vi "Update time.vi"(8 "error in (no error)":errorcluster, 10 "Time Stamp Control":timestamp, 11 "Common Measurements Interface in":refnum<class "Common Measurements Interface.lvclass">) -> (0 "error out":errorcluster, 3 "Common Measurements Interface out":refnum<class "Common Measurements Interface.lvclass">)   [LabVIEW 2015, in "Common Measurements Interface.lvclass"]
uses:
  Common Measurements Interface.lvclass
  Common Measurements Interface.lvclass/Common Measurements Interface.ctl
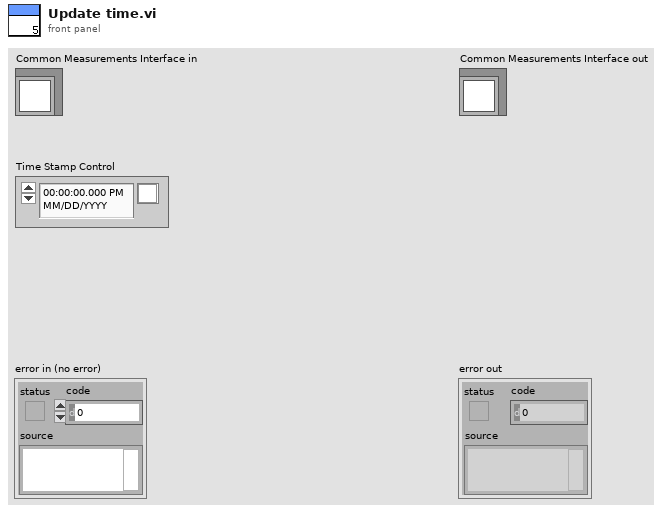
[diagram p1: front panel]
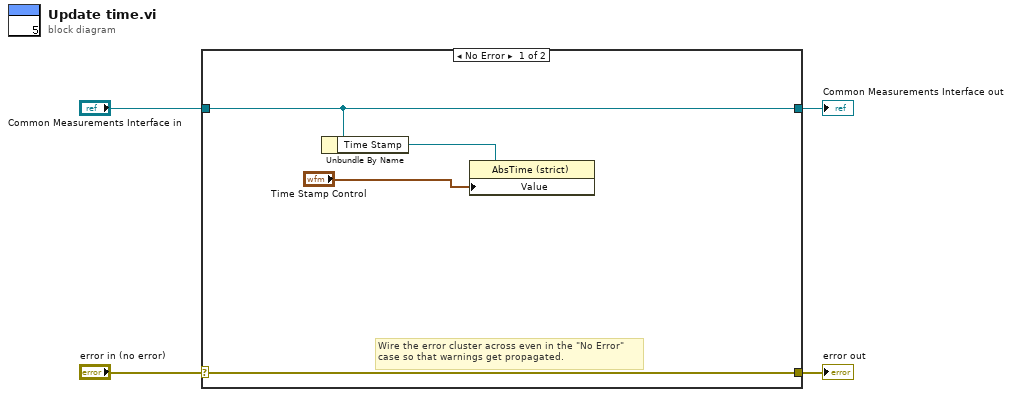
[diagram p0: block diagram]
diagram:
  n1 = case shown="No Error" "error in (no error)" {
    selector: "error in (no error)" -> [w8 w10]
    tunnel: [w8 w10] -> w3
    tunnel: [w7 w9] -> w1
    tunnel: "Common Measurements Interface in" -> [w7 w9]
    frame No Error {
      # "Wire the error cluster across even in the \"No Error\"\ncase so that warnings get propagated."
      n2 = Unbundle By Name(w7) -> ("Time Stamp"=w6:refnum<vi>)
      n3 = property class="AbsTime (strict)"(reference=w6, "Value"="Time Stamp Control") -> ()  [unwired: 1 in, 2 out]
    }
    frame Error {
    }
  }
  "error out" <- w3
  "Common Measurements Interface out" <- w1
